vi "Measurement UI.vi"() -> ()   [LabVIEW 2023, in "FPT_SParam UI.lvlib"]
uses:
  FPT_SParam UI.lvlib
panel:
  in  "Tab Control 2":T1(tab)
  out "General Graph 1":T2(graph)
  out "General Graph 2":T2(graph)
  in  "Power sequencing file validity check":bool
  in  "SnP File Path (String)":string
  in  "Calset File Path (String)":string
  in  "RFmxVNA Port1 s2p file path (String)":string
  in  "RFmxVNA attenuation mode":enum32{"<None>", "s2p File"}(ring)=enum."s2p File"
  in  "RFmxVNA name":string="5842_0"
  in  "Power sequencing file path":string
  in  "RFmxVNA Port2 s2p file path (String)":string
  out "All Graph Refs":refnum<vi>[](array[refnum])
  in  "Measurement S-Parameters":string[](array[combo])
  out "VNA Status":string
  out "S-Param Magnitude":dbl[][](array[numeric])
  out "S-Param Phase":dbl[][](array[numeric])
  out "S-Param":dbl[][](array[numeric])
  out "MeasTable":string[][](table)
  in  "Configuration":T3(ring)
  in  "Tab Control":T4(tab)
  in  "Power sequencing file path_update":path caption="Power Sequencing File Path"
  in  "vCal Name":string
  in  "RFmxVNA Calset Interpolation":bool caption="Interpolation"
  in  "RFmxVNA Calset Enable":bool caption="Enable"
  in  "Calset File Path":path
  in  "RFmx attenuation mode_tab":enum32{"<None>", "s2p File"}(tab) caption="De-embedding"
  in  "RFmxVNA Port2 Power Compensation":bool caption="Power Compensation Enable"
  in  "RFmxVNA Port2 s-parameters orientation":enum32{"Port1 Towards DUT", "Port2 Towards DUT"}(ring) caption="Orientation"
  in  "RFmxVNA Port1 s-parameters orientation":enum32{"Port1 Towards DUT", "Port2 Towards DUT"}(ring) caption="Orientation"
  in  "RFmxVNA Port1 Power Compensation":bool caption="Power Compensation Enable"
  in  "RFmxVNA Port1 s2p file path_update":path caption="Port1 s2p"
  in  "RFmxVNA Port2 s2p file path_update":path caption="Port2 s2p"
  in  "RFmx name_update":refnum<k15> caption="RFmxVNA Name"
  in  "Save S2P Result":path
  in  "Measurement":enum16{"S11", "S21", "S12", "S22"}[](array[ring])
  in  "Number of Points":i32=200
  in  "Start Frequency (Hz)":dbl=4000000000.0 caption="Start Frequency" format="%#pHz"
  in  "Stop Frequency (Hz)":dbl=26000000000.0 caption="Stop Frequency" format="%#pHz"
  in  "Magnitude Units":i32(ring) items=["dB", "Linear"]
  in  "Phase Trace Type":i32(ring) items=["Wrapped", "Unwrapped"]
  in  "Port2 Test Receiver Attenuation (dB)":dbl caption="Port2 Test Receiver Attenuation" format="%#fdB"
  in  "IF Bandwidth (Hz)":dbl=100000.0 caption="IF Bandwidth" format="%#pHz"
  in  "Port2 Power Level (dBm)":dbl=-10.0 caption="Port2 Power Level" format="%#fdBm"
  in  "Port1 Test Receiver Attenuation (dB)":dbl caption="Port1 Test Receiver Attenuation" format="%#fdB"
  in  "Port1 Power Level (dBm)":dbl=-10.0 caption="Port1 Power Level" format="%#fdBm"
  in  "Pulse Acquisition Auto":bool
  in  "Pulse Mode Enabled":bool
  in  "Averaging Enabled":bool
  in  "Averaging Count":u32
  in  "Pulse Period":dbl=0.001 format="%#ps"
  in  "Pulse Modulator Delay":dbl format="%#ps"
  in  "Pulse Modulator Width":dbl=0.0001 format="%#ps"
  in  "Pulse Acquisition Delay":dbl=2e-05 format="%#ps"
  in  "Pulse Acquisition Width":dbl=4.665e-05 format="%#ps"
  in  "Action":enum32{"Calibrate", "Measure"}(ring)=enum."Measure"
  out "Status":string
  # "Calset Correction"
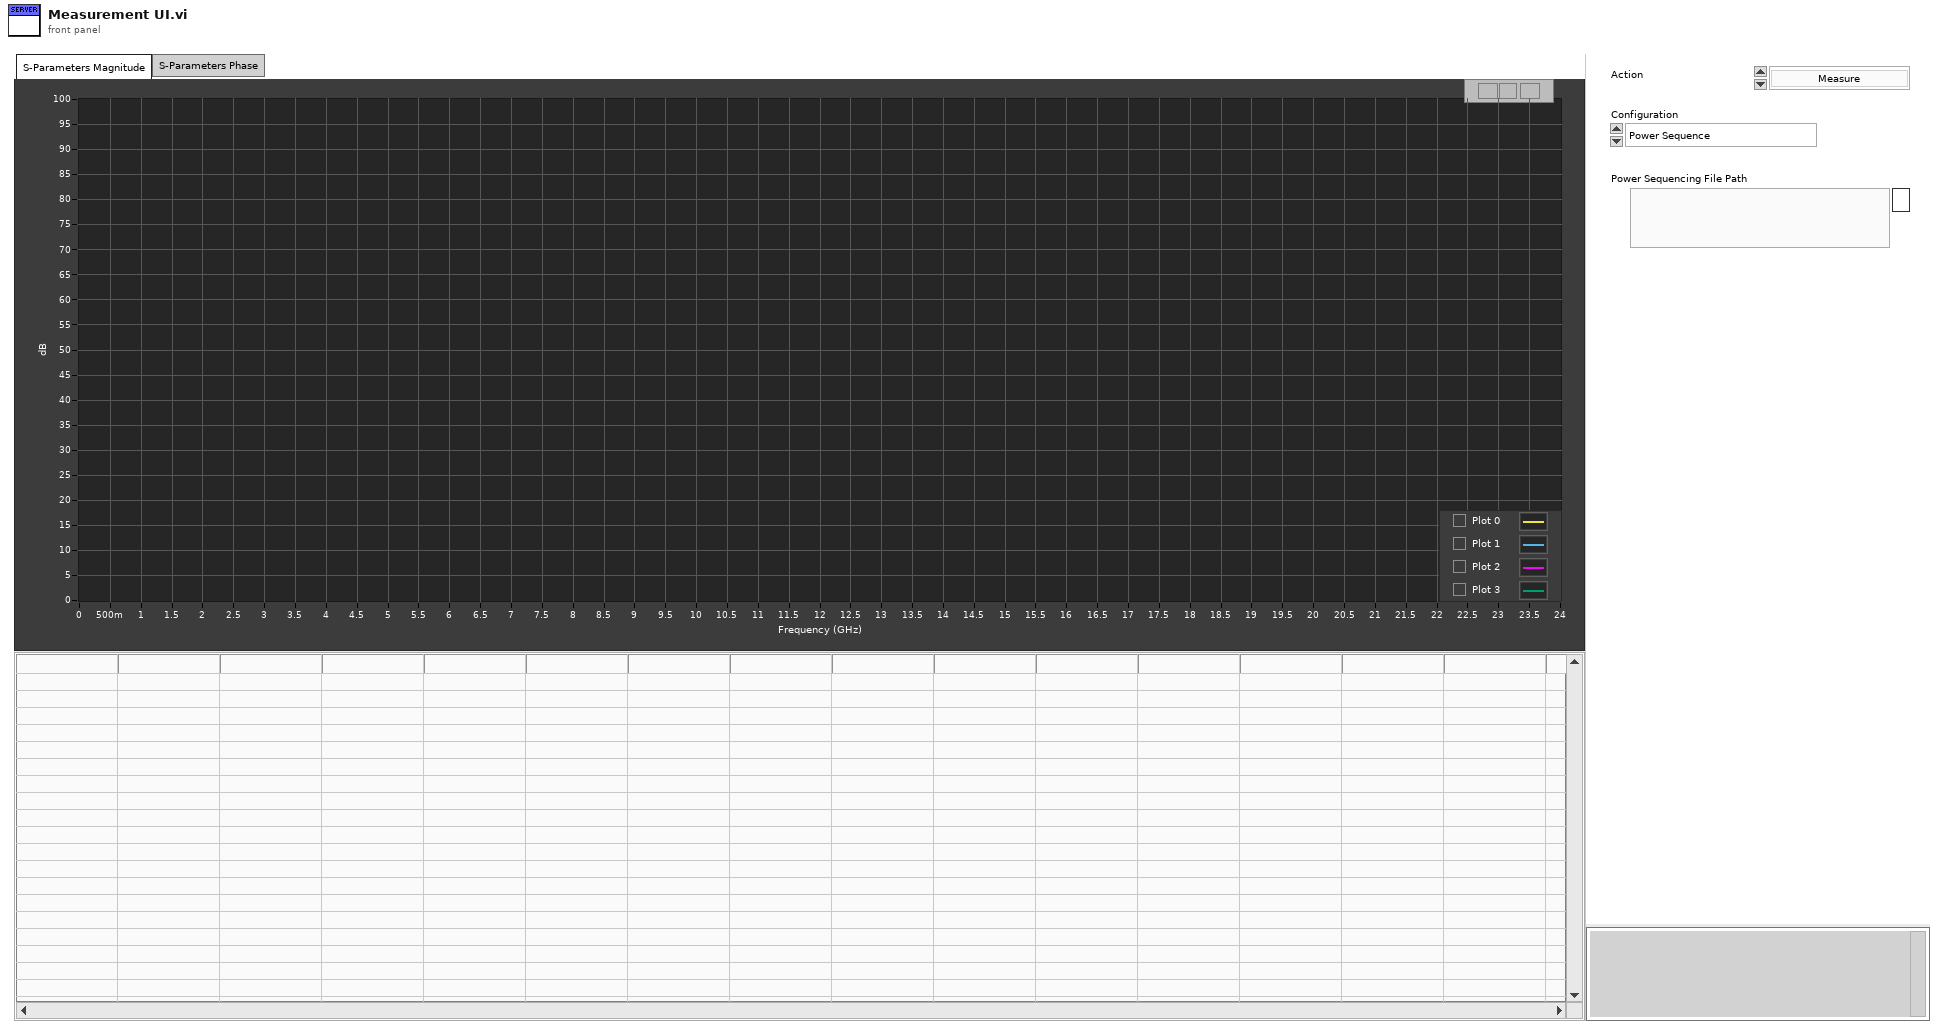
[diagram p1: front panel]
types:
  T1 = enum32{"S-Parameters Magnitude", "S-Parameters Phase", "Hiden Controls"}
  T2 = cluster{"Load currents":dbl[], "Efficiency":dbl[]}[]
  T3 = enum32{"Power Sequence", "HW + Correction", "Measurement 1", "Measurement 2"}
  T4 = enum32{"Power Sequence", "Correction", "Measurement 1", "Measurement 2"}
  T5 = cluster{"Shift":bool, "Ctrl":bool, "Alt":bool, "Cmd":bool, "Opt":bool}
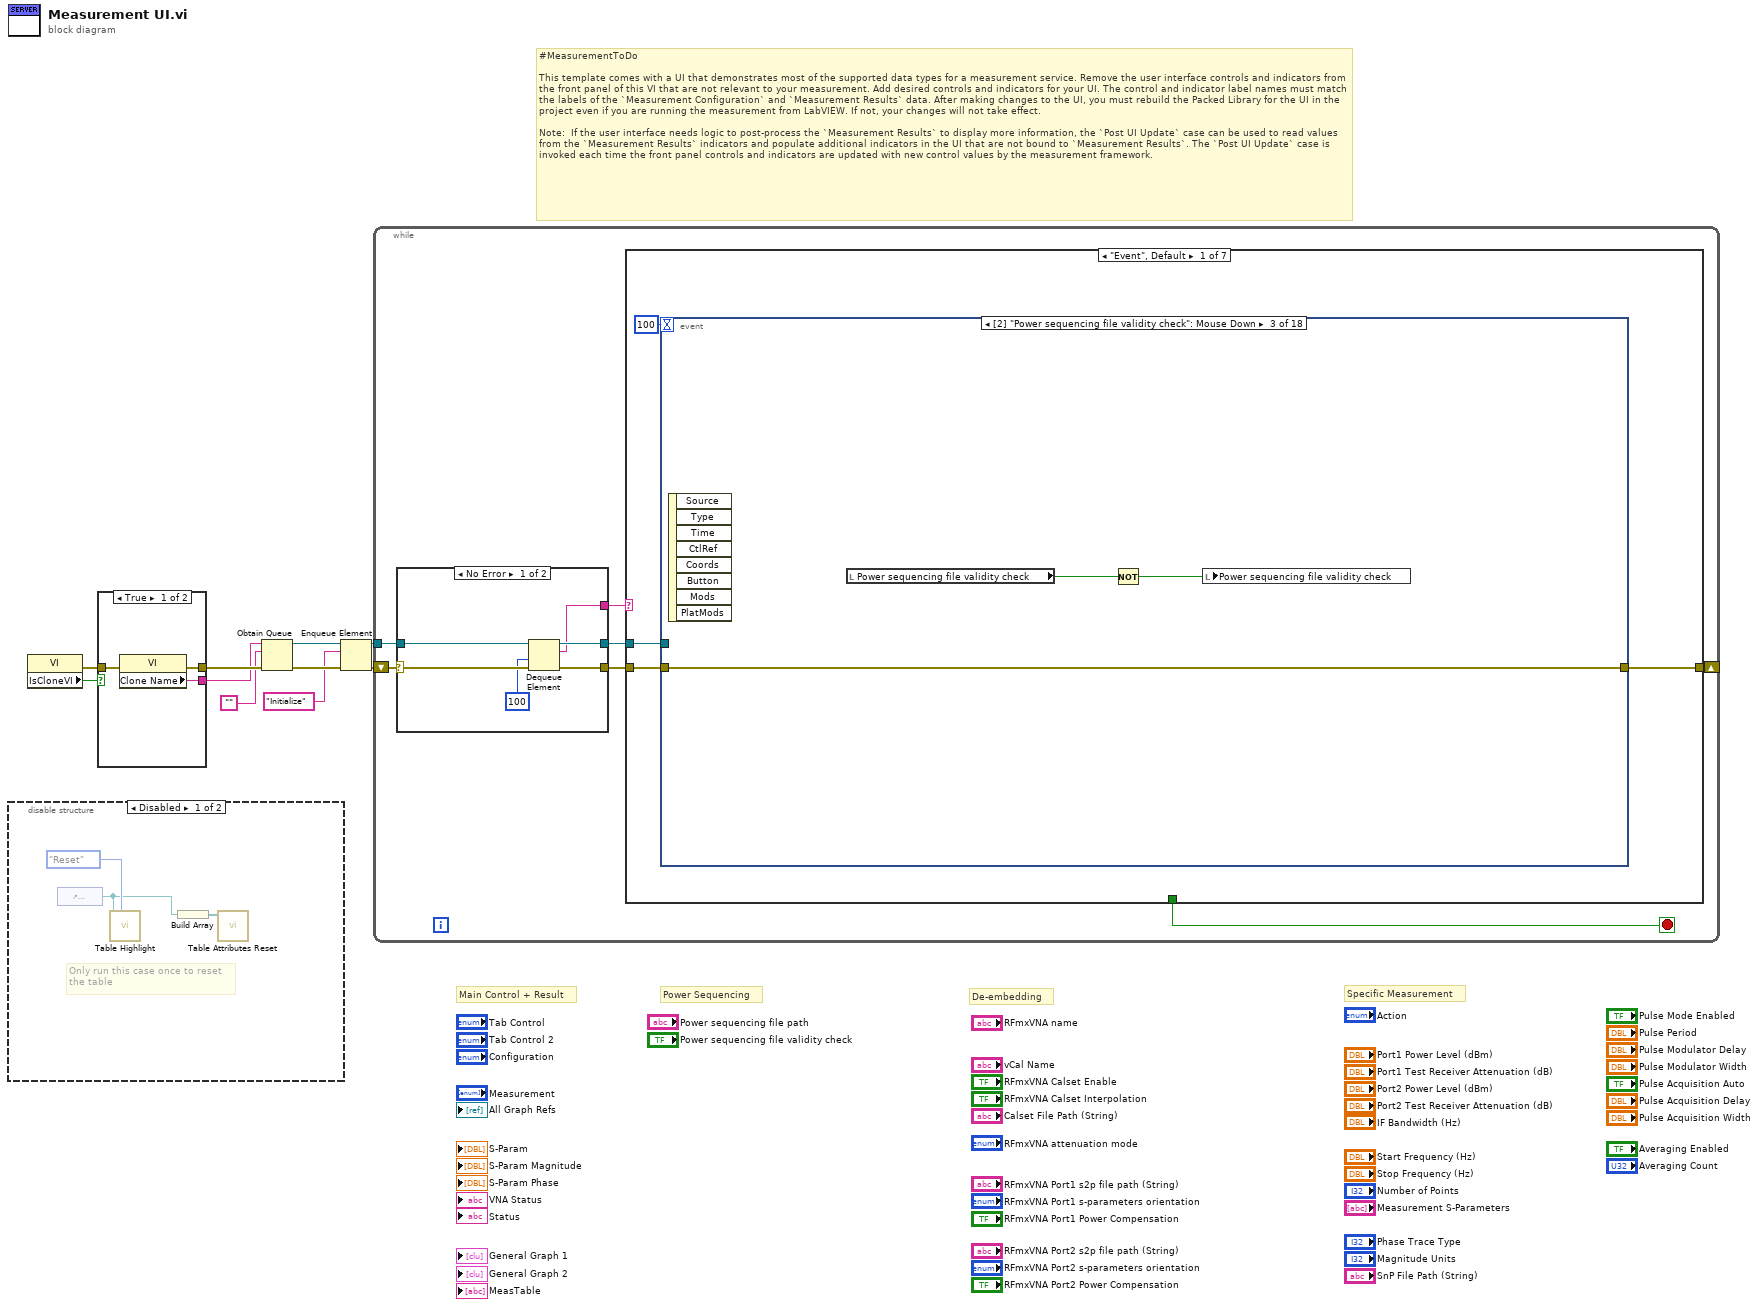
[diagram p0: block diagram]
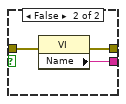
[diagram p3: hidden frame]
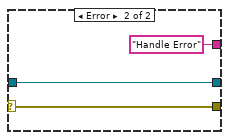
[diagram p4: hidden frame]
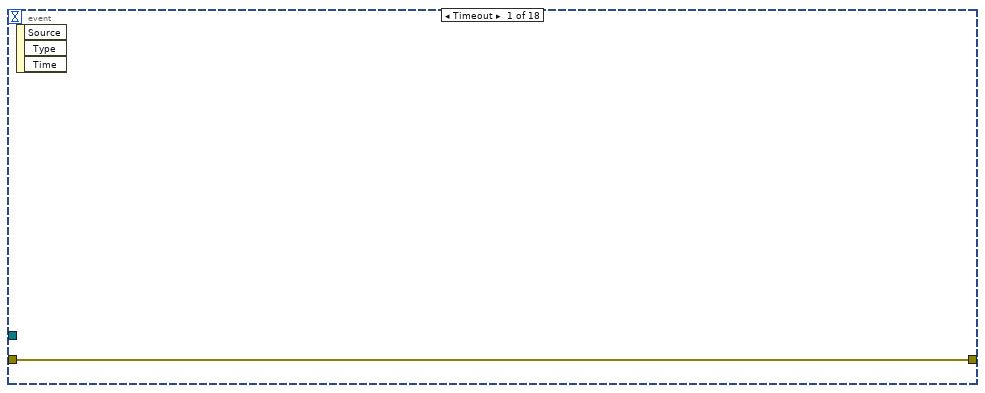
[diagram p5: hidden frame]
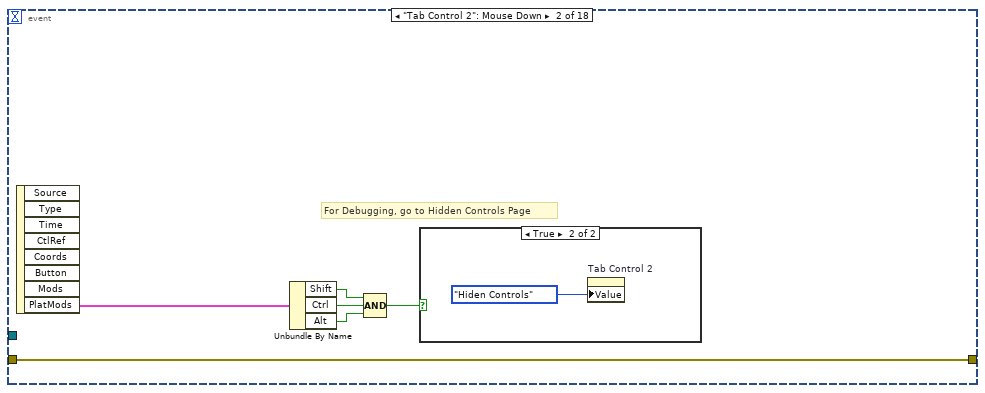
[diagram p6: hidden frame]
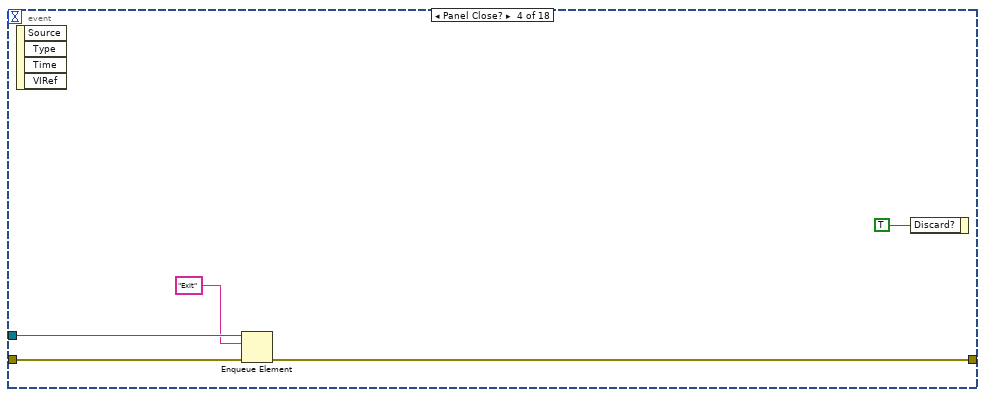
[diagram p8: hidden frame]
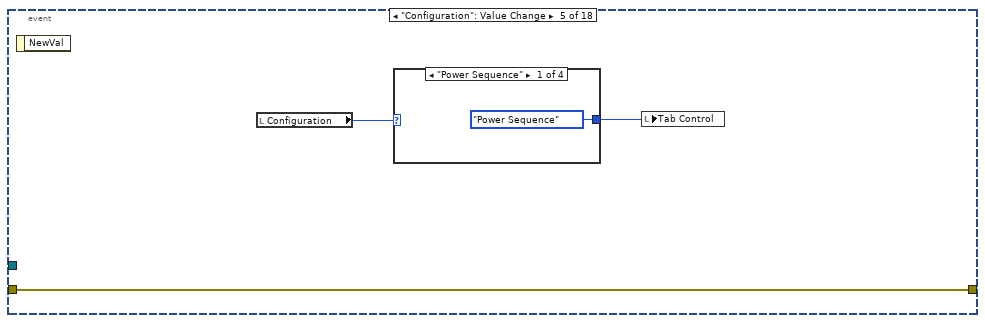
[diagram p9: hidden frame]
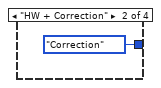
[diagram p10: hidden frame]
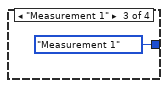
[diagram p11: hidden frame]
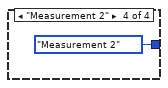
[diagram p12: hidden frame]
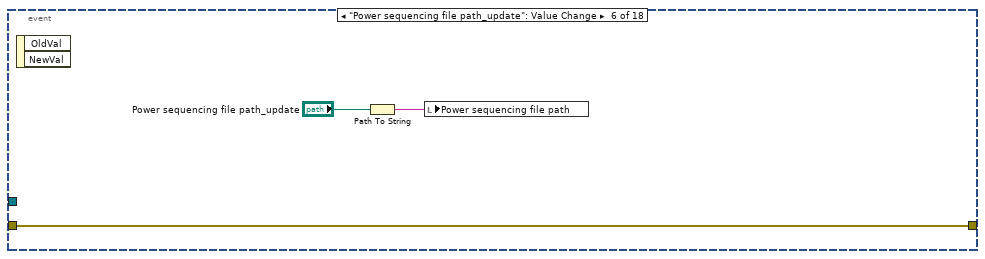
[diagram p13: hidden frame]
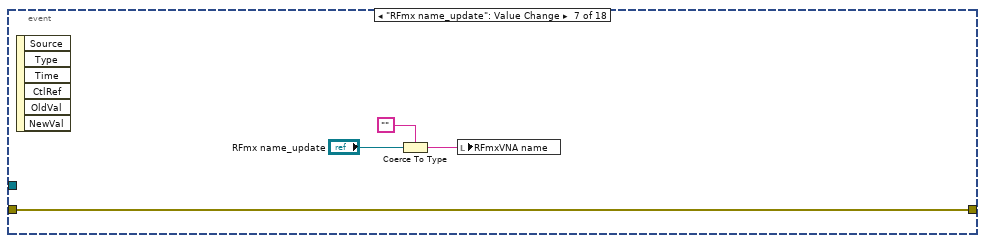
[diagram p14: hidden frame]
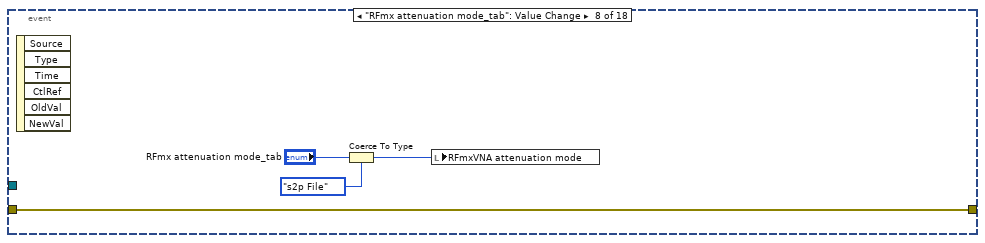
[diagram p15: hidden frame]
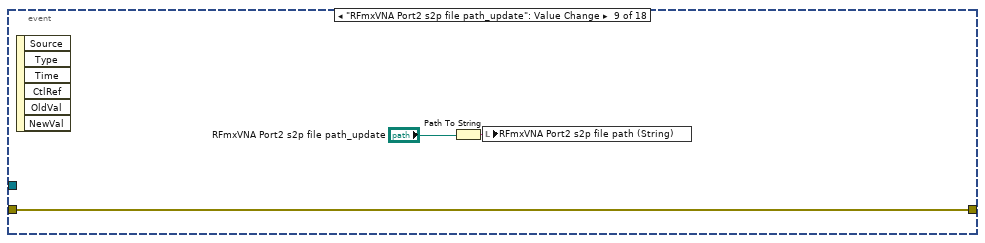
[diagram p16: hidden frame]
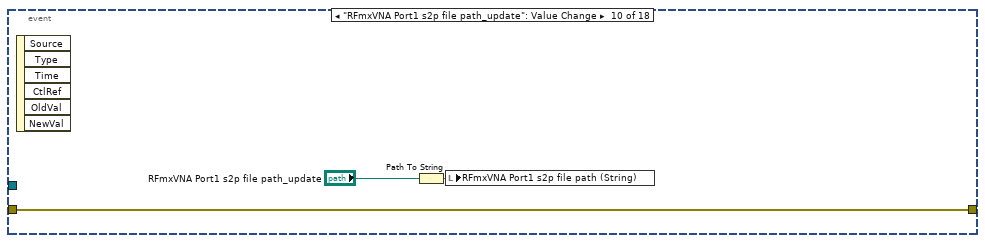
[diagram p17: hidden frame]
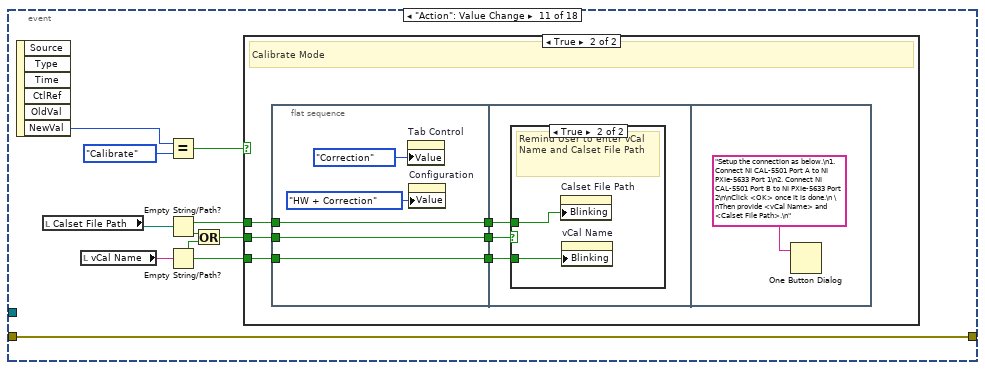
[diagram p18: hidden frame]
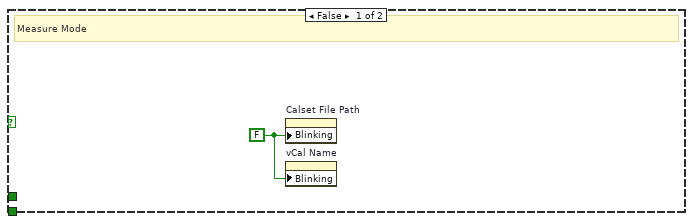
[diagram p19: hidden frame]
diagram:
  # "Specific Measurement"
  # "De-embedding"
  # "Power Sequencing"
  # "Main Control + Result"
  # "#MeasurementToDo  \n\nThis template comes with a UI that demonstrates most of the supported data types for a measurement service. Remove the user interface controls and indicators from the front panel of this VI that are not relevant to your measurement. Add desired controls and indicators for your UI. The control and indicator label names must match the labels of the `Measurement Configuration` and `Measurement Results` data. After making changes to the UI, you must rebuild the Packed Library for the UI in the project even if you are running the measurement from LabVIEW. If not, your changes will not take effect.\n\nNote:  If the user interface needs logic to post-process the `Measurement Results` to display more information, the `Post UI Update` case can be used to read values from the `Measurement Results` indicators and populate additional indicators in the UI that are not bound to `Measurement Results`. The `Post UI Update` case is invoked each time the front panel controls and indicators are updated with new control values by the measurement framework."
  n1 = disable-structure shown="Disabled" {
    frame Disabled {
      # "Only run this case once to reset\nthe table"
      n2 = control-ref of="MeasTable"() -> (w11:refnum<vi>)
      n3 = call "Table Highlight.vi"("Action"=enum16{"Reset", "Highlight 1 Row"}."Reset", "Table Ref in"=w11) -> ()  [unwired: 8 in, 2 out]
      n4 = Build Array(w11) -> (w12:refnum<vi>[])
      n5 = call "Table Attributes Reset.vi"("Table Refs"=w12) -> ()  [unwired: 11 in]
    }
    frame Enabled {
    }
  }
  n6 = property class="VI"() -> (error out=w1:errorcluster, "IsCloneVI"=w2:bool)  [unwired: 2 in, 1 out]
  n7 = case shown="True" w2 {
    tunnel: [w16 w19] -> w10
    tunnel: [w15 w18] -> w9
    tunnel: w1 -> [w14 w17]
    frame True {
      n8 = property class="VI"(error in=w14) -> (error out=w16:errorcluster, "Clone Name"=w15:string)  [unwired: 1 in, 1 out]
    }
    frame False {
      n9 = property class="VI"(error in=w17) -> (error out=w19:errorcluster, "Name"=w18:string)  [unwired: 1 in, 1 out]
    }
  }
  n10 = Obtain Queue(name (unnamed)=w9, element data type="", error in (no error)=w10) -> (queue out=w6:refnum<queue>, error out=w8:errorcluster)  [unwired: 2 in, 1 out]
  n11 = Enqueue Element(queue=w6, element="Initialize", error in (no error)=w8) -> (queue out=w5:refnum<queue>, error out=w7:errorcluster)  [unwired: 1 in, 1 out]
  n12 = while {
    shift-right: [w21] -> _
    shift-left: w7 -> [w26]
    tunnel: w5 -> [w24]
    stop <- w20 stop-if-true
    n13 = case shown="No Error" w26 {
      selector: w26 -> [w32 w35]
      tunnel: [w31 w35] -> w25
      tunnel: w24 -> [w30 w34]
      tunnel: [w29 w34] -> w23
      tunnel: [w28 "Handle Error"] -> w22
      frame No Error {
        n14 = Dequeue Element(queue=w30, timeout in ms (-1)=100, error in (no error)=w32) -> (queue out=w29:refnum<queue>, element=w28:string, error out=w31:errorcluster)  [unwired: 1 out]
      }
      frame Error {
      }
    }
    n15 = case shown="\"Event\", Default" w22 {
      tunnel: w25 -> [w38 w167 w193 w220 w231 w238 w239]
      tunnel: w23 -> [w36 _ w192 w219 _ w236 _]
      tunnel: [w39 w167 w193 w221 w230 w233 w239] -> w21
      tunnel: [_ _ _ _ _ TRUE _] -> w20
      frame "Event", Default {
        n16 = event shown="[2] \"Power sequencing file validity check\": Mouse Down" {
          selector: _ -> [_ _ _ _ _ _ _ _ _ _ _ _ _ _ _ _ _ _]
          dyn-events: _ -> [_ _ _ _ _ _ _ _ _ _ _ _ _ _ _ _ _ _]
          timeout: 100 -> [_ _ _ _ _ _ _ _ _ _ _ _ _ _ _ _ _ _]
          tunnel: [w40 w46 w50 w53 w58 w63 w66 w71 w76 w77 w88 w108 w110 w115 w124 w127 w135 w152] -> w39
          tunnel: w38 -> [w40 w46 w50 w54 w58 w63 w66 w71 w76 w77 w88 w108 w110 w115 w124 w127 w135 w153]
          tunnel: w36 -> [_ _ _ w52 _ _ _ _ _ _ _ _ _ _ _ _ _ _]
          event Timeout {
            n17 = event-data() -> ()  [unwired: 1 in, 3 out]
          }
          event "Tab Control 2": Mouse Down {
            # "For Debugging, go to Hidden Controls Page"
            n18 = event-data() -> ("PlatMods"=w45:T5)  [unwired: 1 in, 7 out]
            n19 = Unbundle By Name(w45) -> ("Shift"=w44:bool, "Ctrl"=w43:bool, "Alt"=w42:bool)
            n20 = Compound Arithmetic op=AND(w44, w43, w42) -> (w41:bool)
            n21 = case shown="True" w41 {
              frame False {
              }
              frame True {
                n22 = property on="Tab Control 2" class="TabCtl (strict)"("Value"=T1."Hiden Controls" ("Tab Control 2")) -> ()  [unwired: 2 in, 2 out]
              }
            }
          }
          event "Power sequencing file validity check": Mouse Down {
            n23 = event-data() -> ()  [unwired: 1 in, 8 out]
            n24 = local read "Power sequencing file validity check"() -> (w49:bool)
            n25 = Not(x=w49) -> (.not. x?=w48:bool)
            n26 = local write "Power sequencing file validity check"(w48) -> ()
          }
          event Panel Close? {
            n27 = event-data() -> ()  [unwired: 1 in, 4 out]
            n28 = Enqueue Element(queue=w52, element="Exit", error in (no error)=w54) -> (error out=w53:errorcluster)  [unwired: 1 in, 2 out]
            n29 = event-data("Discard?"=TRUE) -> ()  [unwired: 1 in, 1 out]
          }
          event "Configuration": Value Change {
            n30 = event-data() -> ()  [unwired: 1 in, 1 out]
            n31 = local read "Configuration"() -> (w56:T3)
            n32 = case shown="\"Power Sequence\"" w56 {
              tunnel: [T4."Power Sequence" ("Tab Control") T4."Correction" ("Tab Control") T4."Measurement 1" ("Tab Control") T4."Measurement 2" ("Tab Control")] -> w57
              frame "Power Sequence" {
              }
              frame "HW + Correction" {
              }
              frame "Measurement 1" {
              }
              frame "Measurement 2" {
              }
            }
            n33 = local write "Tab Control"(w57) -> ()
          }
          event "Power sequencing file path_update": Value Change {
            n34 = event-data() -> ()  [unwired: 1 in, 2 out]
            n35 = Path To String(path="Power sequencing file path_update") -> (string=w64:string)
            n36 = local write "Power sequencing file path"(w64) -> ()
          }
          event "RFmx name_update": Value Change {
            n37 = event-data() -> ()  [unwired: 1 in, 6 out]
            n38 = Coerce To Type(0:"RFmx name_update", 1:"") -> (2:w68:string)
            n39 = local write "RFmxVNA name"(w68) -> ()
          }
          event "RFmx attenuation mode_tab": Value Change {
            n40 = event-data() -> ()  [unwired: 1 in, 6 out]
            n41 = Coerce To Type(0:"RFmx attenuation mode_tab", 1:enum32{"<None>", "s2p File"}."s2p File" ("RFmxVNA attenuation mode")) -> (2:w72:enum32{"<None>", "s2p File"})
            n42 = local write "RFmxVNA attenuation mode"(w72) -> ()
          }
          event "RFmxVNA Port2 s2p file path_update": Value Change {
            n43 = event-data() -> ()  [unwired: 1 in, 6 out]
            n44 = Path To String(path="RFmxVNA Port2 s2p file path_update") -> (string=w75:string)
            n45 = local write "RFmxVNA Port2 s2p file path (String)"(w75) -> ()
          }
          event "RFmxVNA Port1 s2p file path_update": Value Change {
            n46 = event-data() -> ()  [unwired: 1 in, 6 out]
            n47 = Path To String(path="RFmxVNA Port1 s2p file path_update") -> (string=w78:string)
            n48 = local write "RFmxVNA Port1 s2p file path (String)"(w78) -> ()
          }
          event "Action": Value Change {
            n49 = event-data() -> ("NewVal"=w86:enum32{"Calibrate", "Measure"})  [unwired: 1 in, 5 out]
            n50 = local read "Calset File Path"() -> (w84:path)
            n51 = local read "vCal Name"() -> (w87:string)
            n52 = Equal?(x=w86, y=enum32{"Calibrate", "Measure"}."Calibrate") -> (x = y?=w80:bool)
            n53 = Empty String/Path?(string/path=w84) -> (empty?=w82:bool)
            n54 = Empty String/Path?(string/path=w87) -> (empty?=w83:bool)
            n55 = Or(x=w82, y=w83) -> (x .or. y?=w81:bool)
            n56 = case shown="True" w80 {
              tunnel: w83 -> [_ w91]
              tunnel: w82 -> [_ w95]
              tunnel: w81 -> [_ w93]
              frame False {
                w89 = FALSE ("Blinking")
                # "Measure Mode"
                n57 = property on="Calset File Path" class="Path"("Blinking"=w89) -> ()  [unwired: 2 in, 2 out]
                n58 = property on="vCal Name" class="Str"("Blinking"=w89) -> ()  [unwired: 2 in, 2 out]
              }
              frame True {
                # "Calibrate Mode"
                n59 = flat-sequence {
                  tunnel: w95 -> [w100]
                  tunnel: [w100] -> w94
                  tunnel: w93 -> [w99]
                  tunnel: [w99] -> w92
                  tunnel: w91 -> [w98]
                  tunnel: [w98] -> w90
                  tunnel: w94 -> [w102]
                  tunnel: w92 -> [w103]
                  tunnel: w90 -> [w101]
                  frame #0 {
                    n60 = property on="Tab Control" class="TabCtl (strict)"("Value"=T4."Correction" ("Tab Control")) -> ()  [unwired: 2 in, 2 out]
                    n61 = property on="Configuration" class="Enum (strict)"("Value"=T3."HW + Correction" ("Configuration")) -> ()  [unwired: 2 in, 2 out]
                  }
                  frame #1 {
                    n62 = case shown="True" w103 {
                      tunnel: w101 -> [_ w105]
                      tunnel: w102 -> [_ w104]
                      frame False {
                      }
                      frame True {
                        # "Remind User to enter vCal Name and Calset File Path"
                        n63 = property on="Calset File Path" class="Path"("Blinking"=w104) -> ()  [unwired: 2 in, 2 out]
                        n64 = property on="vCal Name" class="Str"("Blinking"=w105) -> ()  [unwired: 2 in, 2 out]
                      }
                    }
                  }
                  frame #2 {
                    n65 = One Button Dialog(message="Setup the connection as below.\n1. Connect NI CAL-5501 Port A to NI PXIe-5633 Port 1\n2. Connect NI CAL-5501 Port B to NI PXIe-5633 Port 2\n\nClick <OK> once it is done.\n \nThen provide <vCal Name> and <Calset File Path>.\n") -> ()  [unwired: 1 in, 1 out]
                  }
                }
              }
            }
          }
          event "vCal Name": Mouse Down {
            n66 = event-data() -> ()  [unwired: 1 in, 8 out]
            n67 = property on="vCal Name" class="Str"("Blinking"=FALSE) -> ()  [unwired: 2 in, 2 out]
          }
          event "Calset File Path": Mouse Down {
            n68 = event-data() -> ()  [unwired: 1 in, 8 out]
            n69 = property on="Calset File Path" class="Path"("Blinking"=FALSE) -> ()  [unwired: 2 in, 2 out]
          }
          event "RFmxVNA Calset Enable": Value Change {
            n70 = event-data() -> ("NewVal"=w111:bool)  [unwired: 1 in, 5 out]
            n71 = local read "Calset File Path"() -> (w114:path)
            n72 = Empty String/Path?(string/path=w114) -> (empty?=w112:bool)
            n73 = And(x=w111, y=w112) -> (x .and. y?=w113:bool)
            n74 = case shown="True" w113 {
              frame False {
              }
              frame True {
                # "Remind User to provide Calset File Path that will be used to save the Cal Data."
                n75 = call "File Dialog"("pattern (all files)"="*.ncst*") -> ("selected path"=w119:path, "cancelled"=w118:bool, "error out"=w116:errorcluster)  [unwired: 11 in, 1 out]
                n76 = case shown="False" w118 {
                  tunnel: w119 -> [w120 _]
                  tunnel: w116 -> [_ _]
                  frame False {
                    n77 = property on="Calset File Path" class="Path"("Val(Sgnl)"=w120) -> ()  [unwired: 2 in, 2 out]
                  }
                  frame True {
                    n78 = property on="RFmxVNA Calset Enable" class="Bool (strict)"("Value"=FALSE ("RFmxVNA Calset Enable")) -> ()  [unwired: 2 in, 2 out]
                  }
                }
              }
            }
          }
          event "Calset File Path": Value Change {
            n79 = event-data() -> ()  [unwired: 1 in, 6 out]
            n80 = Path To String(path="Calset File Path") -> (string=w123:string)
            n81 = local write "Calset File Path (String)"(w123) -> ()
          }
          event "Save S2P Result": Value Change {
            n82 = event-data() -> ()  [unwired: 1 in, 6 out]
            n83 = Path To String(path="Save S2P Result") -> (string=w125:string)
            n84 = local write "SnP File Path (String)"(w125) -> ()
          }
          event "Measurement": Value Change {
            n85 = event-data() -> ()  [unwired: 1 in, 6 out]
            n86 = local read "Measurement"() -> (w134:enum16{"S11", "S21", "S12", "S22"}[])
            n87 = Sort 1D Array(array=w134) -> (sorted array=w128:enum16{"S11", "S21", "S12", "S22"}[])
            n88 = for {
              tunnel: w128 -> [w137] mode=indexing
              tunnel: [w139] -> w131 mode=indexing
              shift-right: [w140] -> w132
              shift-left: variant ("variant") -> [w142]
              n89 = Format Into String(w137) -> (resulting string=w139:string)  [unwired: 3 in, 1 out]
              n90 = Number To Decimal String(number=w137) -> (decimal integer string=w136:string)  [unwired: 1 in]
              n91 = Get Variant Attribute(Variant=w142, name=w136, default value (empty Variant)=w139) -> (duplicate Variant=w141:variant, value=w138:string)  [unwired: 1 in, 2 out]
              n92 = Set Variant Attribute(Variant=w141, name=w136, value=w138) -> (Variant out=w140:variant)  [unwired: 1 in, 2 out]
            }
            n93 = Get Variant Attribute(Variant=w132) -> (values=w129:variant[])  [unwired: 3 in, 3 out]
            n94 = Variant To Data(type=w131, Variant=w129) -> (data=w130:string[])  [unwired: 1 in, 1 out]
            n95 = local write "Measurement S-Parameters"(w130) -> ()
          }
          event "General Graph 1", "General Graph 2": Cursor Move {
            n96 = event-data() -> ("CtlRef"=w143:refnum<vi>, "PointIdx"=w146:i32, "CursLoc"=w151:cluster{"X":dbl, "Y":dbl})  [unwired: 1 in, 6 out]
            n97 = Unbundle By Name(w151) -> ("X"=w150:dbl)
            n98 = property on="All Graph Refs" class="Arr (strict)"() -> ("Value"=w147:refnum<vi>[])  [unwired: 2 in, 2 out]
            n99 = Search 1D Array(1D array=w147, element=w143) -> (index of element=w149:i32)  [unwired: 1 in]
            n100 = Delete From Array(array=w147, index=w149) -> (array with subset deleted=w148:refnum<vi>[])  [unwired: 1 in, 1 out]
            n101 = call "Graph Cursor Update.vi"("Action"=enum16{"Reset", "Update"}."Update" ("Cursor to Update"), "error in"=w153, "New X position"=w150, "Cursor Type"=enum16{"Movable", "Fixed", "All"}."Movable", "Graph Refs in"=w148) -> ("error out"=w156:errorcluster)  [unwired: 5 in, 1 out]
            n102 = control-ref of="MeasTable"() -> (w145:refnum<vi>)
            n103 = call "Table Highlight.vi"("Action"=enum16{"Reset", "Highlight 1 Row"}."Highlight 1 Row", "error in"=w156, "Color Box"=u32 16776960, "Row"=w146, "Table Ref in"=w145) -> ("error out"=w158:errorcluster)  [unwired: 5 in, 1 out]
            n104 = call <vilib>:"Clear Errors.vi"("error in (no error)"=w158, "specific error code to clear (0: all)"=1055) -> ("error out"=w152:errorcluster)  [unwired: 4 in, 1 out]
          }
        }
      }
      frame "Initialize" {
        w160 = enum16{"S11", "S21", "S12", "S22"}[] [enum."S11", enum."S21", enum."S12", enum."S22"] items=["S11", "S21", "S12", "S22"] ("Value (Signaling)")
        w161 = 0
        n105 = control-ref of="General Graph 1"() -> (w165:refnum<vi>)
        n106 = control-ref of="General Graph 2"() -> (w162:refnum<vi>)
        n107 = local write "Tab Control"(w161) -> ()
        n108 = local write "Tab Control 2"(w161) -> ()
        n109 = local write "Configuration"(w161) -> ()
        n110 = local write "Action"(enum32{"Calibrate", "Measure"}."Measure" ("Action")) -> ()
        n111 = Build Array(w165, w162) -> (w164:refnum<vi>[])
        n112 = property on="All Graph Refs" class="Arr (strict)"("Value"=w164) -> ()  [unwired: 2 in, 2 out]
        n113 = call "Graph Set Cursor Mode.vi"("Cursor Mode"=enum32{"Free-Drag", "Single-Plot", "Multi-Plot"}."Multi-Plot", "Graph Refs in"=w164) -> ()  [unwired: 8 in, 2 out]
        n114 = property on="Measurement" class="Arr (strict)"("Val(Sgnl)"=w160) -> ()  [unwired: 2 in, 2 out]
      }
      frame "Post UI Update" {
        # "This case will be triggered, after framework updates the User interface with result values.\nUsed to update data type def"
        n115 = local read "RFmxVNA Port1 s2p file path (String)"() -> (w179:string)
        n116 = local read "RFmxVNA Port2 s2p file path (String)"() -> (w178:string)
        n117 = local read "Power sequencing file path"() -> (w189:string)
        n118 = local read "Calset File Path (String)"() -> (w171:string)
        n119 = local read "SnP File Path (String)"() -> (w169:string)
        n120 = Enqueue Element(queue=w192, element="Post UI Update 2") -> ()  [unwired: 2 in, 3 out]
        n121 = String To Path(string=w171) -> (path=w170:path)
        n122 = String To Path(string=w169) -> (path=w168:path)
        n123 = String To Path(string=w189) -> (path=w190:path)
        n124 = String To Path(string=w179) -> (path=w176:path)
        n125 = String To Path(string=w178) -> (path=w177:path)
        n126 = local read "Measurement S-Parameters"() -> (w172:string[])
        n127 = local write "Power sequencing file path_update"(w190) -> ()
        n128 = local write "RFmxVNA Port1 s2p file path_update"(w176) -> ()
        n129 = local write "RFmxVNA Port2 s2p file path_update"(w177) -> ()
        n130 = local write "Calset File Path"(w170) -> ()
        n131 = local write "Save S2P Result"(w168) -> ()
        n132 = local read "VNA Status"() -> (w175:string)
        n133 = Equal?(x=w175, y="Successfully Calibrated") -> (x = y?=w174:bool)
        n134 = for {
          tunnel: w172 -> [w199] mode=indexing
          tunnel: [w196] -> w181 mode=indexing
          n135 = property on="S-Param 2" class="Enum (strict)"() -> ("Value"=w197:enum16{"S11", "S21", "S12", "S22"}, "Strings []"=w200:string[])  [unwired: 2 in, 2 out]
          n136 = Search 1D Array(1D array=w200, element=w199) -> (index of element=w198:i32)  [unwired: 1 in]
          n137 = Coerce To Type(0:w198, 1:w197) -> (2:w196:enum16{"S11", "S21", "S12", "S22"})
        }
        n138 = case shown="True" w174 {
          selector: w174 -> [_ w195]
          frame False {
          }
          frame True {
            n139 = local write "VNA Status"("" ("VNA Status")) -> ()
            n140 = property on="RFmxVNA Calset Enable" class="Bool (strict)"("Value"=w195) -> ()  [unwired: 2 in, 2 out]
          }
        }
        n141 = local read "RFmxVNA Port1 s2p file path (String)"() -> (w188:string)
        n142 = local read "RFmxVNA name"() -> (w184:string)
        n143 = local read "RFmxVNA attenuation mode"() -> (w182:enum32{"<None>", "s2p File"})
        n144 = Coerce To Type(0:w184, 1:refnum<k15> refnum ("RFSG name_update")) -> (2:w186:refnum<k15>)
        n145 = local write "RFmx name_update"(w186) -> ()
        n146 = Coerce To Type(0:w182, 1:enum32{"<None>", "s2p File"}."s2p File" ("RFmx attenuation mode_tab")) -> (2:w183:enum32{"<None>", "s2p File"})
        n147 = String To Path(string=w188) -> (path=w187:path)
        n148 = local write "RFmxVNA Port1 s2p file path_update"(w187) -> ()
        n149 = local write "RFmx attenuation mode_tab"(w183) -> ()
        n150 = local write "Measurement"(w181) -> ()
      }
      frame "Post UI Update 2" {
        # "Phase Graph"
        # "Mag Graph"
        # "Run after Post UI Update. Can be duplicate is need more processing.\nUtilize this case to convert the result to graph or table"
        n151 = Enqueue Element(queue=w219, element="Post UI Update 3", error in (no error)=w220) -> (error out=w221:errorcluster)  [unwired: 1 in, 2 out]
        n152 = local read "Magnitude Units"() -> (w206:i32)
        n153 = control-ref of="General Graph 1"() -> (w217:refnum<vi>)
        n154 = property on="S-Param Magnitude" class="Arr (strict)"() -> ("Value"=w211:dbl[][])  [unwired: 2 in, 2 out]
        n155 = control-ref of="General Graph 2"() -> (w213:refnum<vi>)
        n156 = property on="S-Param Phase" class="Arr (strict)"() -> ("Value"=w208:dbl[][])  [unwired: 2 in, 2 out]
        n157 = control-ref of="Measurement"() -> (w218:refnum<vi>)
        n158 = call "Get S-Param Names - SParam.vi"("Array in"=w218) -> ("Plot Names"=w212:string[])  [unwired: 10 in]
        n159 = for {
          tunnel: w211 -> [w225] mode=indexing
          tunnel: w208 -> [w224] mode=indexing
          tunnel: [w223] -> w209 mode=concatenating
          n160 = Build Array(w225, w224) -> (w223:dbl[][])
        }
        n161 = call "Graph Assign Plot Names and Data.vi"("Legend Number of Rows"=4, "X Ys Data"=w211, "Plot Names"=w212, "Graph Ref in"=w217) -> ("Graph Ref out"=w205:refnum<vi>)  [unwired: 5 in, 2 out]
        n162 = call "Graph Assign Plot Names and Data.vi"("Legend Number of Rows"=4, "X Ys Data"=w208, "Plot Names"=w212, "Graph Ref in"=w213) -> ()  [unwired: 5 in, 3 out]
        n163 = call "Get Magnitude and Phase Header - SParam.vi"("Magnitude Units"=w206, "x-axis"="Frequency (GHz)" ("S-Parameter"), "Plot Names"=w212) -> ("Header"=w215:string[])  [unwired: 8 in]
        n164 = property on="Magnitude Units" class="Ring (strict)"() -> ("RingText.Text"=w203:string)  [unwired: 2 in, 2 out]
        n165 = control-ref of="MeasTable"() -> (w214:refnum<vi>)
        n166 = Delete From Array(array=w209, index (row)=0 ("index")) -> (array with subset deleted=w207:dbl[][])  [unwired: 2 in, 1 out]
        n167 = call "Table Set Header Name and Data.vi"("Data"=w207, "Header"=w215, "Table Ref"=w214) -> ()  [unwired: 9 in]
        n168 = property class="XYGraph (strict)"(reference=w205, "ActYScl"=0 ("Active Y Scale"), "YScale.NameLbl.Text"=w203) -> ()  [unwired: 1 in, 2 out]
      }
      frame "Post UI Update 3" {
        n169 = property on="All Graph Refs" class="Arr (strict)"() -> ("Value"=w227:refnum<vi>[])  [unwired: 2 in, 2 out]
        n170 = call "Graph Cursor Update.vi"("Action"=enum16{"Reset", "Update"}."Update", "error in"=w231, "New X position"=0.0, "Cursor Type"=enum16{"Movable", "Fixed", "All"}."Movable", "Graph Refs in"=w227) -> ("error out"=w230:errorcluster)  [unwired: 5 in, 1 out]
      }
      frame "Exit" {
        # "This case is triggered to close the User Interface from framework"
        n171 = Flush Queue(queue=w236, error in (no error)=w238) -> (queue out=w235:refnum<queue>, error out=w234:errorcluster)  [unwired: 1 out]
        n172 = Release Queue(queue=w235, force destroy? (F)=TRUE, error in (no error)=w234) -> (error out=w233:errorcluster)  [unwired: 2 out]
      }
      frame "Handle Error" {
      }
    }
  }
